vi "Actor Core.vi"(8 "error in":errorcluster, 11 "Calibration Actor in":refnum<class "Calibration Actor.lvclass">) -> (0 "error out":errorcluster, 3 "Actor out":refnum<class "Actor.lvclass">)   [LabVIEW 2014, in "Calibration.lvlib" / "Calibration Actor.lvclass"]
doc: "(<B>Filename</B>: Actor Framework.lvlib:Actor.lvclass:Actor Core.vi)\n\nReceives messages to the actor, reacts to them, and initiates any error handling that may shut the actor down.\n\nDescendant classes may override this VI to append parallel tasks for the actor to complete while it handles messages. Overrides use the Call Parent Method node."
uses:
  Calibration Actor.lvclass
  <vilib>/ActorFramework/Actor/Actor.lvclass
  Calibration Actor.lvclass/Calibration Actor.ctl
  SuperActor/Ex Nested.lvclass
  reusable/Sequence/SEQ/SEQ.lvclass
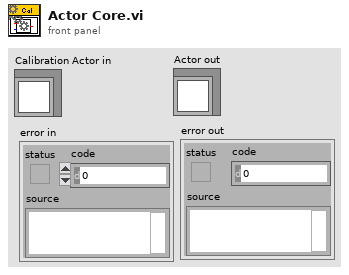
[diagram p1: front panel]
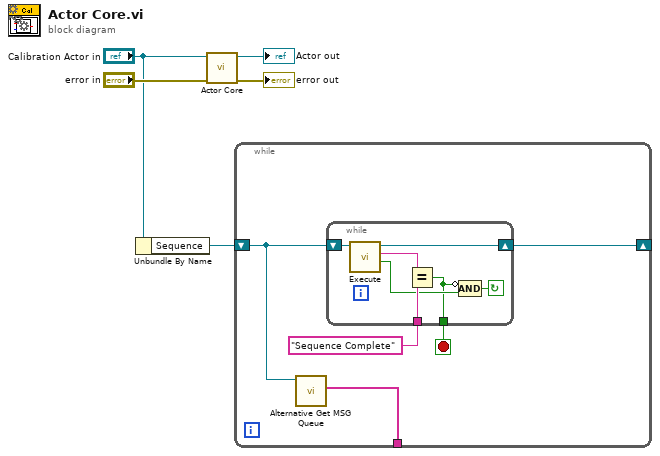
[diagram p0: block diagram]
diagram:
  n1 = Unbundle By Name("Calibration Actor in") -> ("Sequence"=w1:refnum<class "SEQ.lvclass">)
  n2 = call-parent "Actor Core.vi"("error in"="error in", "Actor in"="Calibration Actor in") -> ("error out"=→"error out":errorcluster, "Actor out"=→"Actor out":refnum<class "Actor.lvclass">)  [unwired: 8 in]
  n3 = while {
    shift-right: [w9] -> _
    shift-left: w1 -> [w7]
    tunnel: [w6] -> _
    stop <- w8 stop-if-true
    n4 = call "Alternative Get MSG Queue.vi"("SEQ in"=w7) -> ("seqMsg"=w6:string[])  [unwired: 9 in, 1 out]
    n5 = while {
      shift-right: [w17] -> w9
      shift-left: w7 -> [w16]
      tunnel: "Sequence Complete" ("y") -> [w14]
      tunnel: [w11] -> w8
      stop <- w12 continue-if-true
      n6 = call-dynamic "Execute.vi"("SEQ in"=w16) -> ("Next Step?"=w13:bool, "MSG"=w15:string, "SEQ out"=w17:refnum<class "SEQ.lvclass">)  [unwired: 7 in, 1 out]
      n7 = Equal?(x=w15, y=w14) -> (x = y?=w11:bool)
      n8 = Compound Arithmetic op=AND(invert w11, w13) -> (w12:bool)
    }
  }
